vi "Input leakage currents and offset voltage.vi"(0 "数组输入":dbl[](array[numeric])) -> (4 "Voffset":dbl, 6 "Iin-":dbl, 8 "Iin+":dbl, 10 "Iin_mean":dbl, 15 "Iin_bias":dbl)   [LabVIEW 2019]
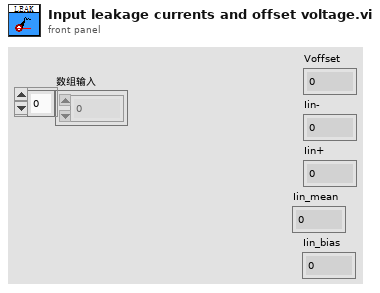
[diagram p1: front panel]
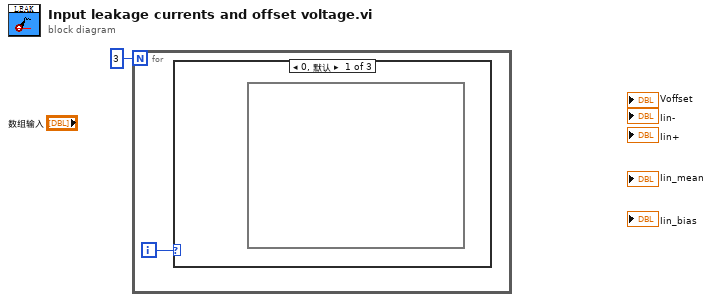
[diagram p0: block diagram]
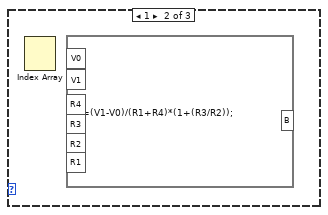
[diagram p2: hidden frame]
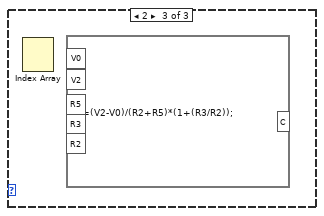
[diagram p3: hidden frame]
diagram:
  n1 = for {
    N: 3 -> [_]
    i -> [w2]
    n2 = case shown="0, 默认" w2 {
      frame 0, Default {
        n3 = formula code=""() -> ()
      }
      frame 1 {
        n4 = Index Array() -> ()  [unwired: 3 in, 2 out]
        n5 = formula code="B=(V1-V0)/(R1+R4)*(1+(R3/R2));"() -> ("B"=w3:dbl)  [unwired: 6 in]
      }
      frame 2 {
        n6 = Index Array() -> ()  [unwired: 3 in, 2 out]
        n7 = formula code="C=(V2-V0)/(R2+R5)*(1+(R3/R2));"() -> ("C"=w4:dbl)  [unwired: 5 in]
      }
    }
  }
